vi "Digital Output Global.vi"() -> ()   [LabVIEW 2023]
panel:
  in  "Number of Channels Parameter Name":string="Number of Channels"
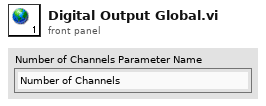
[diagram p1: front panel]
diagram:
